vi "Door Open Interlock Value Change.vi"(8 "error in (no error)":errorcluster, 10 "Door Open Interlock":bool, 11 "Doors Closing in":refnum<class "Doors Closing.lvclass">) -> (0 "error out":errorcluster, 3 "Doors Closing out":refnum<class "Doors Closing.lvclass">)   [LabVIEW 2020, in "Door Controller.lvlib" / "Doors Closing.lvclass"]
uses:
  Doors Closing.lvclass
  C:/Users/Thomas.McQuillan/Desktop/Elevator Door Control/Door Controller/Door Controller/Door Controller.lvclass
  Application/Application/Interlock Names.ctl
  Door Controller/Door Controller.lvclass
  Application/Application.lvlib
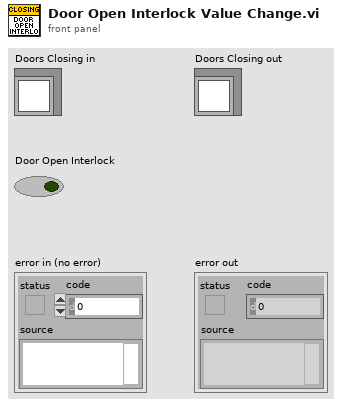
[diagram p1: front panel]
types:
  T1 = typedef "Application.lvlib/Interlock Names.ctl" = enum16{"Door Closed Interlock", "Door Open Interlock"}
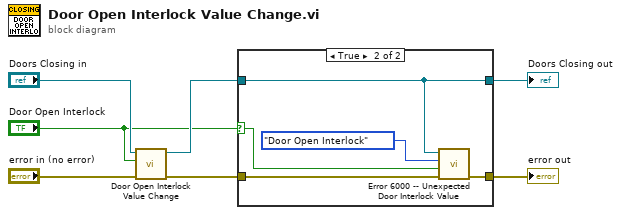
[diagram p0: block diagram]
diagram:
  n1 = call-parent "Door Open Interlock Value Change.vi"("error in (no error)"="error in (no error)", "Door Open Interlock"="Door Open Interlock", "Door Controller in"="Doors Closing in") -> ("error out"=w2:errorcluster, "Door Controller out"=w5:refnum<class "Doors Closing.lvclass">)  [unwired: 7 in]
  n2 = case shown="True" "Door Open Interlock" {
    selector: "Door Open Interlock" -> [_ w13]
    tunnel: w5 -> [w9 w10]
    tunnel: [w9 w10] -> w4
    tunnel: [w8 w11] -> w1
    tunnel: w2 -> [w8 w12]
    frame False {
    }
    frame True {
      n3 = call "Error 6000 -- Unexpected Door Interlock Value.vi"("error in (no error)"=w12, "Interlock Value"=w13, "Interlock Name"=Interlock_Names."Door Open Interlock", "Door Controller"=w10) -> ("error out"=w11:errorcluster)  [unwired: 7 in]
    }
  }
  "error out" <- w1
  "Doors Closing out" <- w4
